vi "Actor Core.vi"(8 "error in":errorcluster, 11 "Nested in":refnum<class "Contador.lvclass">) -> (0 "error out":errorcluster, 3 "Actor out":refnum<class "Actor.lvclass">)   [LabVIEW 2020, in "Contador.lvlib" / "Contador.lvclass"]
doc: "(<B>Filename</B>: Actor Framework.lvlib:Actor.lvclass:Actor Core.vi)\n\nReceives messages to the actor, reacts to them, and initiates any error handling that may shut the actor down.\n\nDescendant classes may override this VI to append parallel tasks for the actor to complete while it handles messages. Overrides use the Call Parent Method node."
uses:
  Contador.lvclass
  Contador.lvclass/Contador.ctl
  <vilib>/ActorFramework/Actor/Actor.lvclass
  <vilib>/ActorFramework/Stop Msg/Stop Msg.lvclass
  Contador Messages/Decrement Msg/Decrement Msg.lvclass
  Contador Messages/Increment Msg/Increment Msg.lvclass
  Contador Messages/Reset Msg/Reset Msg.lvclass
  C:/Program Files (x86)/National Instruments/LabVIEW 2020/vi.lib/ActorFramework/Actor/Actor.lvclass
  D:/Storage/Source Code/Clase AF/ClaseAF/03 AF/Contador/Contador.lvclass
  Contador Messages/update time Msg/update time Msg.lvclass
panel:
  out "Fecha":timestamp format="%<%x %.1X>T"
  in  "Reset":bool
  in  "Decrement":bool
  in  "Increment":bool
  out "Cuenta":dbl format="Cuenta: %.2f"
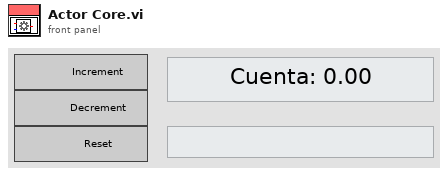
[diagram p1: front panel]
types:
  T1 = cluster{"Stop":refnum<user-event>, "Cuenta":refnum<user-event>, "Fecha":refnum<user-event>}
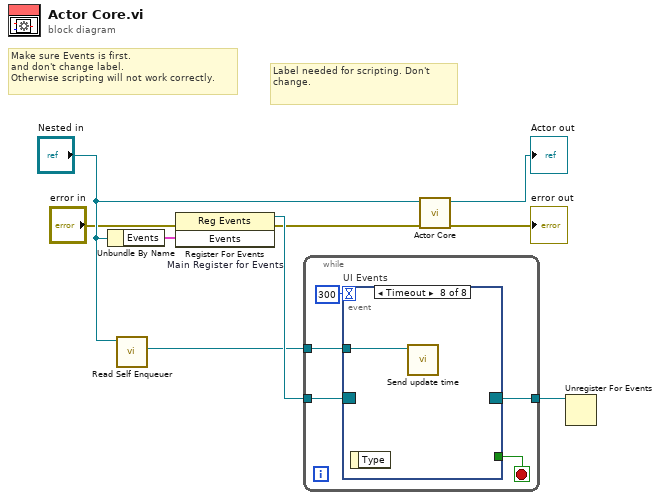
[diagram p0: block diagram]
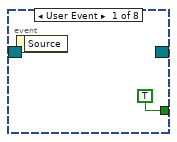
[diagram p2: hidden frame]
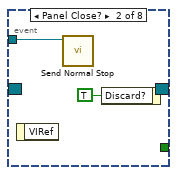
[diagram p3: hidden frame]
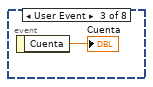
[diagram p4: hidden frame]
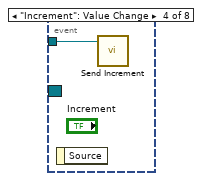
[diagram p5: hidden frame]
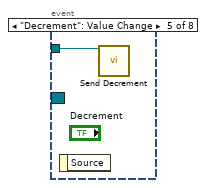
[diagram p6: hidden frame]
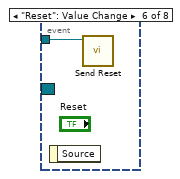
[diagram p7: hidden frame]
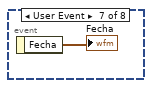
[diagram p8: hidden frame]
diagram:
  # "Label needed for scripting. Don't change."
  # "Make sure Events is first.\nand don't change label.\nOtherwise scripting will not work correctly."
  n1 = Unbundle By Name("Nested in") -> ("Events"=w6:T1)
  n2 = call <vilib>:"Read Self Enqueuer.vi"("Actor"="Nested in") -> ("Self Enqueuer"=w3:refnum<class "Message Enqueuer.lvclass">)  [unwired: 10 in]
  n3 = register-events "Main Register for Events"(error in="error in", w6) -> (reference out=w7:refnum<event-registration>, error out=w1:errorcluster)  [unwired: 1 in]
  n4 = while {
    tunnel: w7 -> [w14]
    tunnel: [w12] -> w5
    tunnel: w3 -> [w11]
    stop <- w13 stop-if-true
    n5 = event "UI Events" shown="[7] Timeout" {
      selector: w14 -> [_ _ _ _ _ _ _ _]
      dyn-events: [_ _ _ _ _ _ _ _] -> w12
      timeout: 300 -> [_ _ _ _ _ _ _ _]
      tunnel: [TRUE _ _ _ _ _ _ _] -> w13
      tunnel: w11 -> [_ w16 _ w19 w20 w21 _ w23]
      event User Event {
        n6 = event-data() -> ()  [unwired: 1 in, 1 out]
      }
      event Panel Close? {
        n7 = event-data() -> ()  [unwired: 1 in, 1 out]
        n8 = call <vilib>:"Send Normal Stop.vi"("Message Enqueuer"=w16) -> ()  [unwired: 10 in, 1 out]
        n9 = event-data("Discard?"=TRUE) -> ()  [unwired: 1 in, 1 out]
      }
      event User Event {
        n10 = event-data() -> ("Cuenta"=→"Cuenta":dbl)  [unwired: 1 in]
      }
      event "Increment": Value Change {
        n11 = event-data() -> ()  [unwired: 1 in, 1 out]
        n12 = call "Send Increment.vi"("Message Enqueuer"=w19) -> ()  [unwired: 9 in, 2 out]
      }
      event "Decrement": Value Change {
        n13 = event-data() -> ()  [unwired: 1 in, 1 out]
        n14 = call "Send Decrement.vi"("Message Enqueuer"=w20) -> ()  [unwired: 9 in, 2 out]
      }
      event "Reset": Value Change {
        n15 = event-data() -> ()  [unwired: 1 in, 1 out]
        n16 = call "Send Reset.vi"("Message Enqueuer"=w21) -> ()  [unwired: 9 in, 2 out]
      }
      event User Event {
        n17 = event-data() -> ("Fecha"=→"Fecha":timestamp)  [unwired: 1 in]
      }
      event Timeout {
        n18 = event-data() -> ()  [unwired: 1 in, 1 out]
        n19 = call "Send update time.vi"("Message Enqueuer"=w23) -> ()  [unwired: 9 in, 2 out]
      }
    }
  }
  n20 = call-parent "Actor Core.vi"("error in"=w1, "Actor in"="Nested in") -> ("error out"=→"error out":errorcluster, "Actor out"=→"Actor out":refnum<class "Actor.lvclass">)  [unwired: 8 in]
  n21 = Unregister For Events(event registration refnum=w5) -> ()  [unwired: 1 in, 1 out]
